vi "Analog Tachometer Process Global.vi"() -> ()   [LabVIEW 2024, in "Analog Tachometer Process.lvlib" / "Analog Tachometer Process.lvclass"]
uses:
  Analog Tachometer Process.lvclass
panel:
  in  "Command":string="Help"
  in  "Positions Unique Channel Identifier":string="Positions"
  in  "Default Positions Channel Name":string="Positions"
  in  "Positions Channel Unit":string="s"
  in  "Samples/Rev Unique Channel Identifier":string="Samples per Revolution"
  in  "Default Samples/Rev Channel Name":string="Samples per Revolution"
  in  "Samples/Rev Channel Unit":string="samples/rev"
  in  "Pulse width Param Default Value":i32=2
  in  "Pulse width Param Name":string="Pulse width"
  in  "Slope Enum Param Current Value":string="Rising"
  in  "Slope Param Name":string="Slope"
  in  "Slope Enum Param Possible Values":string[](array[string])=["Rising", "Falling"]
  in  "Hysteresis Param Default Value":dbl
  in  "Hysteresis Param Name":string="Hysteresis"
  in  "Threshold Param Default Value":dbl
  in  "Threshold Param Name":string="Threshold"
  in  "Pulse/revolution Param Default Value":i32=1
  in  "Current Speed Unique Channel Identifier":string="RPM"
  in  "Pulse/revolution Param Name":string="Pulse/revolution"
  in  "Default Current Speed Channel Name":string="Current Speed"
  in  "Current Speed Channel Unit":string="RPM"
  in  "Select Channel Param Name":string="Select Channel"
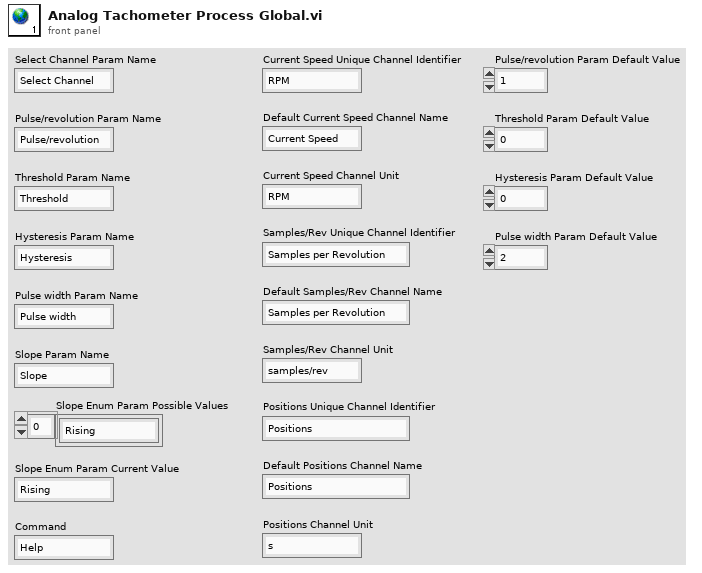
[diagram p1: front panel]
diagram:
